vi "Configure Frequency Coupling.vi"(5 "Coupling Enable (T: Enable)":bool=TRUE, 6 "Coupling Ratio (1)":dbl=1.0, 7 "Coupling Offset (0 Hz)":dbl format="%#.4f", 8 "error in (no error)":errorcluster, 9 "Coupling Mode (1: Ratio)":i32(ring)=1 items=["Offset", "Ratio"], 10 "Channel (1: 1)":i32(ring)=1 items=["1"=1, "2"=2], 11 "VISA resource name":refnum<visa-resource-name>) -> (0 "error out":errorcluster, 3 "VISA resource name out":refnum<visa-resource-name>)   [LabVIEW 2019, in "Agilent 3352X Series.lvlib"]
doc: "Configures frequency coupling between channels. \n\n<b>Note</b>:\n(1) Both channels must be configured to nonArbitrary waveform in order to enable frequency coupling. \n(2) This VI is only valid on a 2-channel instrument."
uses:
  Agilent 3352X Series.lvlib
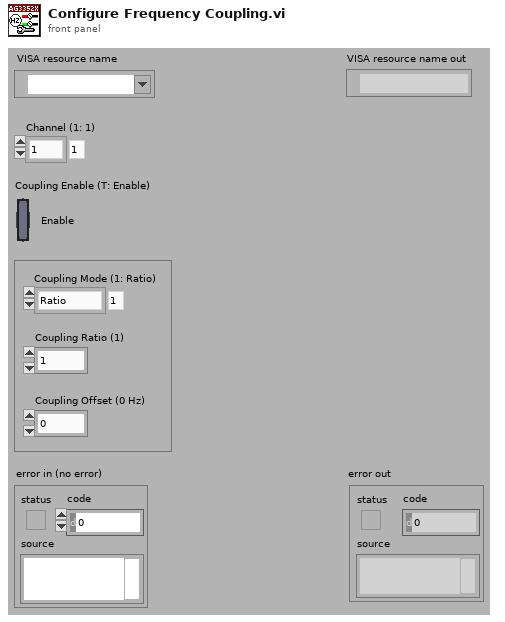
[diagram p1: front panel]
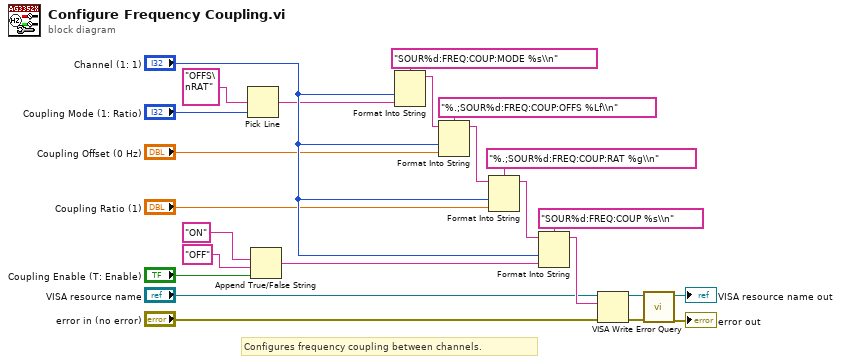
[diagram p0: block diagram]
diagram:
  # "Configures frequency coupling between channels."
  n1 = Pick Line(multi-line string="OFFS\nRAT", line index="Coupling Mode (1: Ratio)") -> (output string=w1:string)  [unwired: 1 out]
  n2 = Append True/False String(1:"Coupling Enable (T: Enable)", 2:"OFF", 3:"ON") -> (0:w11:string)  [unwired: 1 out]
  n3 = Format Into String(format string="SOUR%d:FREQ:COUP:MODE %s\\n", "Channel (1: 1)", w1) -> (resulting string=w22:string)  [unwired: 2 in, 1 out]
  n4 = Format Into String(format string="%.;SOUR%d:FREQ:COUP:OFFS %Lf\\n", initial string=w22, "Channel (1: 1)", "Coupling Offset (0 Hz)") -> (resulting string=w19:string)  [unwired: 1 in, 1 out]
  n5 = Format Into String(format string="%.;SOUR%d:FREQ:COUP:RAT %g\\n", initial string=w19, "Channel (1: 1)", "Coupling Ratio (1)") -> (resulting string=w13:string)  [unwired: 1 in, 1 out]
  n6 = Format Into String(format string="SOUR%d:FREQ:COUP %s\\n", initial string=w13, "Channel (1: 1)", w11) -> (resulting string=w10:string)  [unwired: 1 in, 1 out]
  n7 = VISA Write(VISA resource name="VISA resource name", write buffer=w10, error in (no error)="error in (no error)") -> (VISA resource name out=w7:refnum<visa-resource-name>, error out=w6:errorcluster)  [unwired: 1 out]
  n8 = call "Error Query.vi"("error in (no error)"=w6, "VISA resource name"=w7) -> ("error out"=→"error out":errorcluster, "VISA resource name out"=→"VISA resource name out":refnum<visa-resource-name>)  [unwired: 8 out]
